vi "Tell Self Init.vi"(7 "Actor in":refnum<class "Actor.lvclass">, 8 "Error in":errorcluster, 10 "Input":T1) -> (0 "Error out":errorcluster, 5 "Actor out":refnum<class "Actor.lvclass">)   [LabVIEW 2020, in "_Template.lvlib" / "Templates.lvlib" / "TEMPLATE jettl Msg.lvlib"]
uses:
  TEMPLATE jettl Msg.lvlib
  jettl/jettl/Actor/Actor.lvclass
  Input.ctl
panel:
  # "This front panel should not be manipulated."
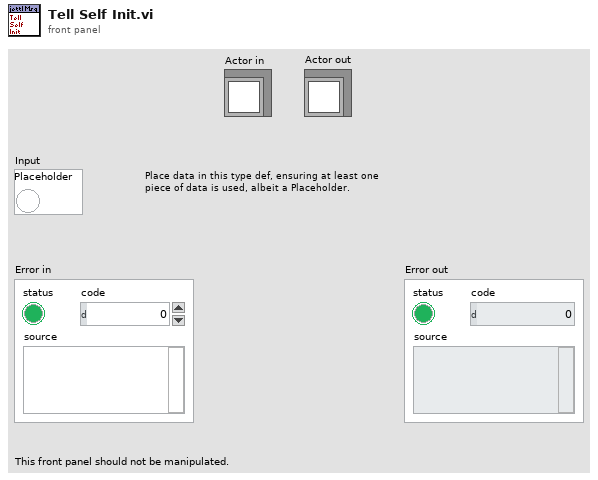
[diagram p1: front panel]
types:
  T1 = typedef "_Template.lvlib/Templates.lvlib/TEMPLATE jettl Msg.lvlib/Input.ctl" = cluster{"Placeholder":bool}
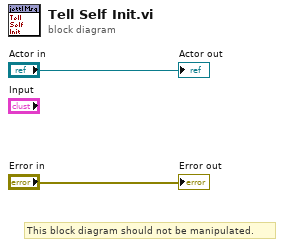
[diagram p0: block diagram]
diagram:
  # "This block diagram should not be manipulated."
  "Error out" <- "Error in"
  "Actor out" <- "Actor in"
